vi "Set Output Frequency.vi"(8 "error in (no error)":errorcluster, 9 "Synchronous":bool, 10 "Frequency":dbl format="%#_6p", 11 "RP Instrument in":refnum<class "RP Instrument.lvclass">) -> (0 "error out":errorcluster, 2 "Actual frequency":dbl format="%#_6pHz", 3 "RP Instrument out":refnum<class "RP Instrument.lvclass">)   [LabVIEW 2019, in "RP Instrument.lvclass"]
uses:
  RP Instrument.lvclass
  RP Command.ctl
  RP Config Offsets.ctl
  RP Status Offsets.ctl
  RP Instrument.lvclass/RP Instrument.ctl
  RP Communicator/RP Communicator.lvclass
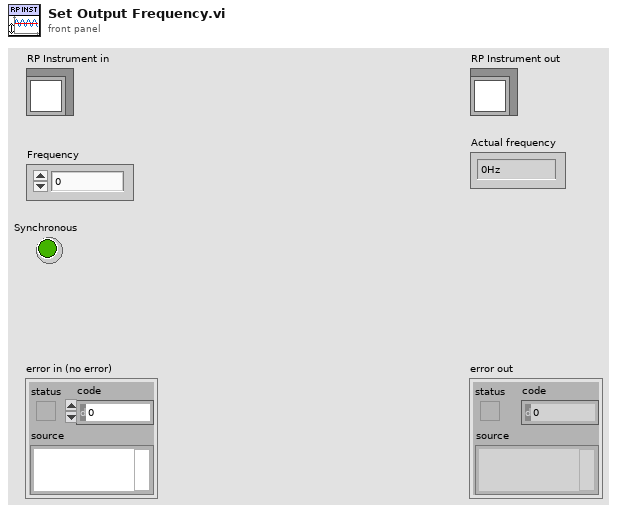
[diagram p1: front panel]
types:
  T1 = typedef "RP Command.ctl" = enum16{"Reset", "Read IDN", "Stop server", "Get status", "Get temperature", "Connect client", "Arm", "Software trigger", "Get whole buffer", "Get chunk", "System call", "Get config", "Set config", "Recieve data", "Recieve Calibartion", "Transmit data"}
  T2 = typedef "RP Status Offsets.ctl" = u16
  T3 = typedef "RP Config Offsets.ctl" = u16
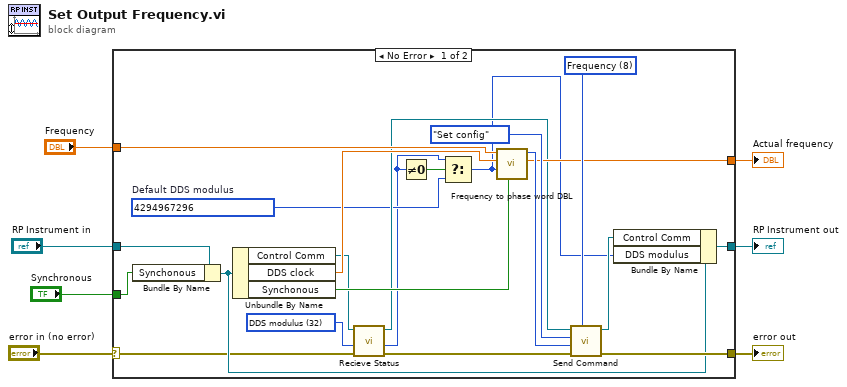
[diagram p0: block diagram]
diagram:
  n1 = case shown="No Error" "error in (no error)" {
    selector: "error in (no error)" -> [w12 w31]
    tunnel: [w27 w31] -> w6
    tunnel: [w26 w30] -> w4
    tunnel: "RP Instrument in" -> [w29 w30]
    tunnel: "Frequency" -> [w22 _]
    tunnel: [w21 _] -> w2
    tunnel: "Synchronous" -> [w17 _]
    frame No Error {
      w10 = i64 4294967296  # Default DDS modulus
      w14 = T2 32 items=["Writer address"=0, "Record start position"=4, "Trig state and ID"=8, "Phase"=12, "X1"=16, "Y1"=20, "RxFIFO counter or  X2"=24, "TxFIFO counter or Y2"=28, "DDS modulus"=32] ("Status offsets")
      w24 = T3 8 items=["Config flags"=0, "Record length"=4, "Frequency"=8, "Decimation"=12, "LED"=16, "DDS delay"=28] ("Config offset")
      n2 = Bundle By Name(cluster=w29, "Synchonous"=w17) -> (w18:refnum<class "RP Instrument.lvclass">)
      n3 = Unbundle By Name(w18) -> ("Control Comm"=w16:refnum<class "RP Communicator.lvclass">, "DDS clock"=w20:dbl, "Synchonous"=w19:bool)
      n4 = call-dynamic "Recieve Status.vi"("error in (no error)"=w12, "Status offset"=w14, "RP Communicator in"=w16) -> ("error out"=w13:errorcluster, "Status response"=w9:u32, "RP Communicator out"=w15:refnum<class "RP Communicator.lvclass">)  [unwired: 6 in]
      n5 = Not Equal To 0?(x=w9) -> (x != 0?=w11:bool)
      n6 = Select(t=w9, s=w11, f=w10) -> (s? t:f=w8:i64)
      n7 = call "Frequency to phase word DBL.vi"("Synchonous"=w19, "DDS modulus"=w8, "DDS clock"=w20, "Frequency"=w22) -> ("Actual frequency"=w21:dbl, "Phase word"=w23:u64)  [unwired: 6 in]
      n8 = call-dynamic "Send Command.vi"("Config offset"=w24, "error in (no error)"=w13, "Command payload"=w23, "Command number"=RP_Command."Set config", "RP Communicator in"=w15) -> ("error out"=w27:errorcluster, "RP Communicator out"=w25:refnum<class "RP Communicator.lvclass">)  [unwired: 5 in]
      n9 = Bundle By Name(cluster=w18, "Control Comm"=w25, "DDS modulus"=w8) -> (w26:refnum<class "RP Instrument.lvclass">)
    }
    frame Error {
    }
  }
  "error out" <- w6
  "RP Instrument out" <- w4
  "Actual frequency" <- w2
